vi "Functiongenerator_control.vi"(2 "error in (no error)":errorcluster, 3 "Data in":string="0 0.5 1000 0 0 2 0 0 0") -> (0 "error out (no error)":errorcluster, 1 "Data Out":string)   [LabVIEW 2011]
doc: "Function Generator VI\nControls a function generator."
uses:
  Server_Globals.vi
panel:
  in  "Duty Cycle High":dbl
  out "User waveform data":dbl[](array[numeric]) format="%.2f"
  in  "Burst count":i32=15
  in  "trigger source":T1(ring)=enum."External" caption="Trigger Source"
  in  "trigger mode":T2(ring)=enum."Stepped" caption="Trigger Mode"
  in  "Waveform":T3(ring)=enum."Square"
  out "Graph":dbl[](graph) caption="User waveform Graph"
  in  "Channel name":string="0"
  in  "Start phase":dbl format="%.2f"
  in  "DC Offset":dbl format="%.2f"
  in  "Amplitude":dbl=0.5 format="%.2f"
  in  "Frequency":dbl=10000.0 format="%.2f"
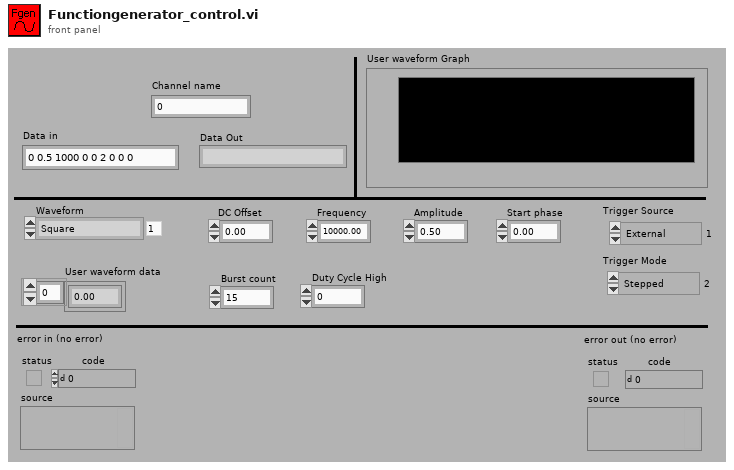
[diagram p1: front panel]
types:
  T1 = enum16{"Immediate", "External", "Software Trigger VI", "GPIB Get", "TTL0", "TTL1", "TTL2", "TTL3", "TTL4", "TTL5", "TTL6", "TTL7", "ECL0", "ECL1", "PXI Star", "RTSI 0", "RTSI 1", "RTSI 2", "RTSI 3", "RTSI 4", "RTSI 5", "RTSI 6"}
  T2 = enum16{"Single", "Continuous", "Stepped", "Burst"}
  T3 = enum16{"Sine", "Square", "Triangle", "Ramp up", "Ramp down", "DC", "Noise", "User Defined"}
  T4 = cluster{"I/O Settings":u64[], "Instrument Handle":cluster{"5402":refnum<k15>, " 5112":refnum<k15>, "4072":refnum<k15>, "USB":refnum<visa-resource-name>, "4110":refnum<k15>}, "Logfile":refnum<file>, "Log Level":i8, "Clear":i32[], "OS Set":cluster{"instrument handle out":refnum<k15>, "remaining string":string, "Settings":cluster{"Horizontal Conf.":cluster{"Min. Sample rate":dbl, "Reference position":dbl, "Record Length":i16}, "Channel A":cluster{"Enable":bool, "Vertical coupling":dbl, "Vertical range":dbl, "Vertical offset":dbl, "Probe attenuation":dbl}, "Channel B":cluster{"Enable":bool, "Vertical coupling":dbl, "Vertical range":dbl, "Vertical offset":dbl, "Probe attenuation":dbl}, "Trigger":cluster{"Source":enum8{"channel 1", "channel 2", "Imediate", "External trigger"}, "Slope":enum8{"Positive", "Negative"}, "Coupling":enum8{"AC", "DC"}, "Level":dbl, "Holdoff":dbl, "Delay":dbl, " Timeout":dbl, " Mode":enum8{"Normal", "Auto", "Auto Level"}}, "Measurements":cluster{"Measurement 1, Channel":enum8{"Channel 1", "Channel 2", "Channel 3", "Channel 4"}, "Measurement 1, Selection":u16, "Measurement 2, Channel":enum8{"Channel 1", "Channel 2", "Channel 3", "Channel 4"}, "Measurement 2,  Selection":u16, "Measurement 3, Channel":enum8{"Channel 1", "Channel 2", "Channel 3", "Channel 4"}, "Measurement 3, Selection 3":u16}}}, "DC Power Supply":cluster{"0":refnum<k15>, "1":refnum<k15>, "2":refnum<k15>, "3":refnum<k15>, "4":refnum<k15>}, "USB Interface":cluster{"0":refnum<visa-resource-name>, "1":refnum<visa-resource-name>, "2":refnum<visa-resource-name>, "3":refnum<visa-resource-name>, "4":refnum<visa-resource-name>}, "Function Generator":cluster{"0":refnum<k15>, "1":refnum<k15>, "2":refnum<k15>, "3":refnum<k15>, "4":refnum<k15>}, "Digital Multimeter":cluster{"0":refnum<k15>, "1":refnum<k15>, "2":refnum<k15>, "3":refnum<k15>, "4":refnum<k15>}, "Digital Osciliscope":cluster{"0":refnum<k15>, "1":refnum<k15>, "2":refnum<k15>, "3":refnum<k15>, "4":refnum<k15>}, "To M Server":string, "Adres":string[][], "Matrix version":string, "MD5":string, "Digital Multimeter Card 2":cluster{"0":string, "1":string, "2":string, "3":string, "4":string}}
  T5 = cluster{"0":refnum<k15>, "1":refnum<k15>, "2":refnum<k15>, "3":refnum<k15>, "4":refnum<k15>}
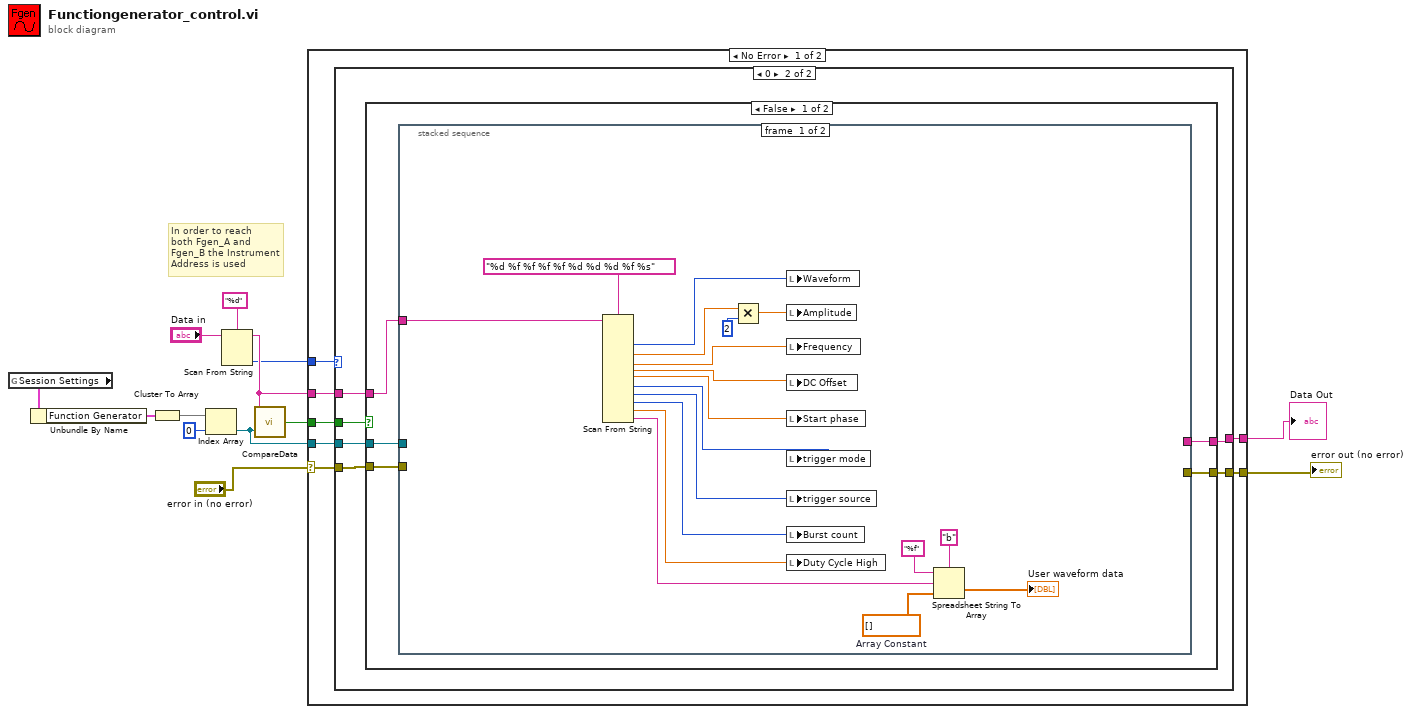
[diagram p0: block diagram]
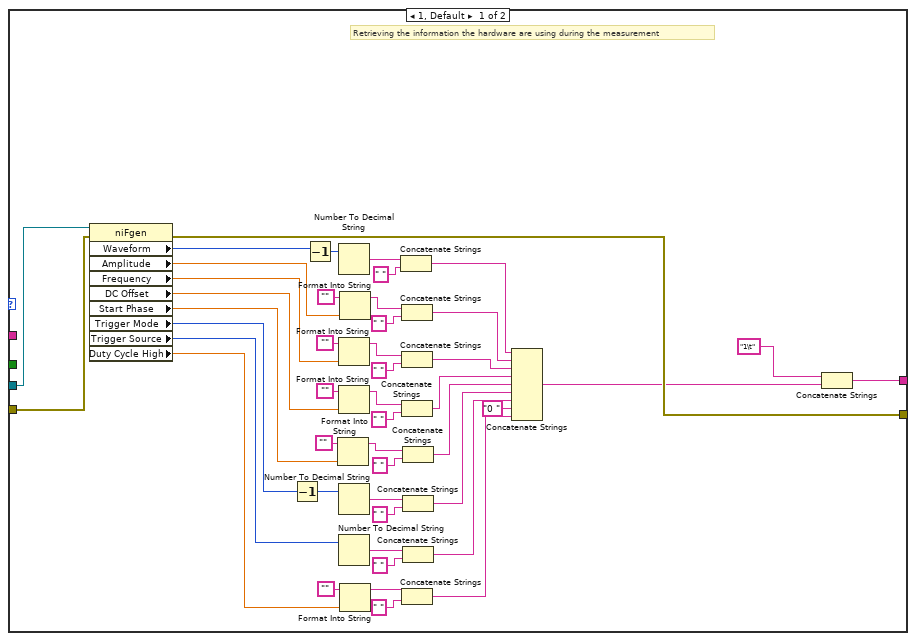
[diagram p2: hidden frame]
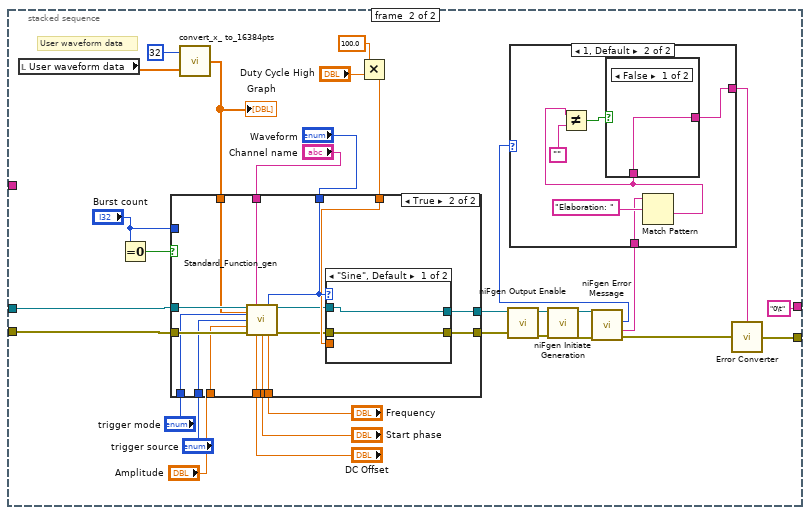
[diagram p3: hidden frame]
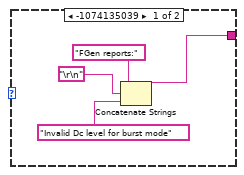
[diagram p4: hidden frame]
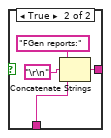
[diagram p5: hidden frame]
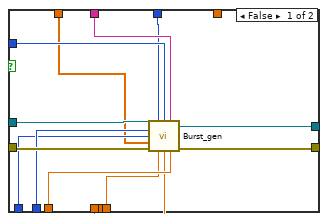
[diagram p6: hidden frame]
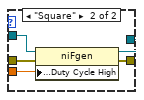
[diagram p7: hidden frame]
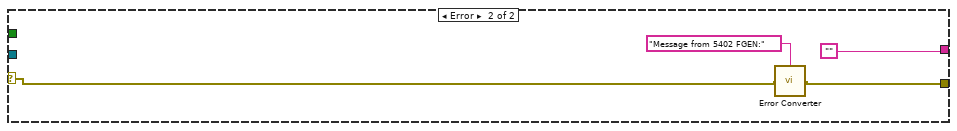
[diagram p9: hidden frame]
diagram:
  # "In order to reach \nboth Fgen_A and \nFgen_B the Instrument\nAddress is used"
  n1 = global read "Server_Globals.vi" "Session Settings"() -> (w5:T4)
  n2 = Unbundle By Name(w5) -> ("Function Generator"=w4:T5)
  n3 = Cluster To Array(cluster=w4) -> (array=w3:refnum<k15>[])
  n4 = Index Array(array=w3, index=0) -> (element=w1:refnum<k15>)
  n5 = Scan From String(format string="%d", input string="Data in") -> (remaining string=w10:string, output 1=w9:i32)  [unwired: 3 in, 2 out]
  n6 = call "CompareData.vi"("Que Name"=w1, "Data input"=w10) -> ("Same as before"=w13:bool)
  n7 = case shown="No Error" "error in (no error)" {
    selector: "error in (no error)" -> [w15 w181]
    tunnel: w13 -> [w20 _]
    tunnel: w1 -> [w19 _]
    tunnel: w10 -> [w18 _]
    tunnel: w9 -> [w17 _]
    tunnel: [w16 w180] -> w8
    tunnel: [w14 ""] -> w6
    frame No Error {
      n8 = case shown="0" w17 {
        tunnel: w20 -> [_ w72]
        tunnel: w18 -> [_ w71]
        tunnel: w19 -> [w29 w70]
        tunnel: w15 -> [w27 w69]
        tunnel: [w26 w68] -> w16
        tunnel: [w23 w67] -> w14
        frame 1, Default {
          # "Retrieving the information the hardware are using during the measurement"
          n9 = property class="niFgen"(reference=w29, error in=w27) -> (error out=w26:errorcluster, "Waveform"=w63:i32, "Amplitude"=w44:dbl, "Frequency"=w39:dbl, "DC Offset"=w36:dbl, "Start Phase"=w34:dbl, "Trigger Mode"=w24:i32, "Trigger Source"=w53:i32, "Duty Cycle High"=w30:dbl)  [unwired: 1 out]
          n10 = Decrement(x=w24) -> (x-1=w25:i32)
          n11 = Decrement(x=w63) -> (x-1=w66:i32)
          n12 = Format Into String(initial string="", w34) -> (resulting string=w33:string)  [unwired: 2 in, 1 out]
          n13 = Number To Decimal String(number=w66) -> (decimal integer string=w65:string)  [unwired: 1 in]
          n14 = Format Into String(initial string="", w39) -> (resulting string=w40:string)  [unwired: 2 in, 1 out]
          n15 = Format Into String(initial string="", w36) -> (resulting string=w37:string)  [unwired: 2 in, 1 out]
          n16 = Number To Decimal String(number=w25) -> (decimal integer string=w57:string)  [unwired: 1 in]
          n17 = Number To Decimal String(number=w53) -> (decimal integer string=w55:string)  [unwired: 1 in]
          n18 = Format Into String(initial string="", w44) -> (resulting string=w42:string)  [unwired: 2 in, 1 out]
          n19 = Format Into String(initial string="", w30) -> (resulting string=w31:string)  [unwired: 2 in, 1 out]
          n20 = Concatenate Strings(w65, " ") -> (w52:string)
          n21 = Concatenate Strings(w42, " ") -> (w51:string)
          n22 = Concatenate Strings(w40, " ") -> (w50:string)
          n23 = Concatenate Strings(w37, " ") -> (w49:string)
          n24 = Concatenate Strings(w31, " ") -> (w45:string)
          n25 = Concatenate Strings(w33, " ") -> (w48:string)
          n26 = Concatenate Strings(w57, " ") -> (w47:string)
          n27 = Concatenate Strings(w55, " ") -> (w46:string)
          n28 = Concatenate Strings(w52, w51, w50, w49, w48, w47, w46, "0 ", w45) -> (w22:string)
          n29 = Concatenate Strings("1\t", w22) -> (w23:string)
        }
        frame 0 {
          n30 = case shown="False" w72 {
            tunnel: w71 -> [w77 _]
            tunnel: w70 -> [w76 _]
            tunnel: w69 -> [w75 w178]
            tunnel: [w74 w178] -> w68
            tunnel: [w73 "0\t"] -> w67
            frame False {
              n31 = stacked-sequence {
                tunnel: w77 -> [w81 _]
                tunnel: w76 -> [_ w125]
                tunnel: w75 -> [_ w124]
                tunnel: [_ w123] -> w74
                tunnel: [_ "0\t"] -> w73
                frame #0 {
                  w94 = dbl[] []  # Array Constant
                  n32 = Scan From String(format string="%d %f %f %f %f %d %d %d %f %s" ("Format String"), input string=w81) -> (output 1=w90:i32, output 2=w83:dbl, output 3=w89:dbl, output 4=w88:dbl, output 5=w87:dbl, output 6=w86:i32, output 7=w85:i32, output 8=w80:i32, output 9=w78:dbl, output 10=w79:string)  [unwired: 12 in, 3 out]
                  n33 = Multiply(x=w83, y=2) -> (x*y=w84:dbl)
                  n34 = local write "Waveform"(w90) -> ()
                  n35 = local write "Amplitude"(w84) -> ()
                  n36 = local write "Frequency"(w89) -> ()
                  n37 = local write "DC Offset"(w88) -> ()
                  n38 = local write "Start phase"(w87) -> ()
                  n39 = local write "trigger mode"(w86) -> ()
                  n40 = local write "trigger source"(w85) -> ()
                  n41 = local write "Burst count"(w80) -> ()
                  n42 = local write "Duty Cycle High"(w78) -> ()
                  n43 = Spreadsheet String To Array(delimiter (Tab)="b", format string="%f", spreadsheet string=w79, array type (2D Dbl)=w94) -> (array=→"User waveform data":dbl[])
                }
                frame #1 {
                  # "User waveform data"
                  n44 = local read "User waveform data"() -> (w106:dbl[])
                  n45 = Equal To 0?(x="Burst count") -> (x = 0?=w108:bool)
                  n46 = call "convert_x_ to_16384pts.vi"("User waveform data"=w106, "Convert_Factor"=32) -> ("Waveform out"=w96:dbl[])
                  "Graph" <- w96
                  n47 = Multiply(x=100.0, y="Duty Cycle High") -> (x*y=w100:dbl)
                  n48 = case shown="True" w108 {
                    tunnel: w125 -> [w153 w169]
                    tunnel: w124 -> [w152 w168]
                    tunnel: [w151 w156] -> w118
                    tunnel: [w150 w157] -> w117
                    tunnel: "Channel name" -> [w149 w167]
                    tunnel: "trigger mode" -> [w147 w166]
                    tunnel: "trigger source" -> [w148 w165]
                    tunnel: "Amplitude" -> [w146 w164]
                    tunnel: "Start phase" -> [_ w160]
                    tunnel: "DC Offset" -> [w145 w162]
                    tunnel: "Frequency" -> [w144 w161]
                    tunnel: "Waveform" -> [w142 w159]
                    tunnel: w96 -> [w141 w163]
                    tunnel: "Burst count" -> [w143 _]
                    tunnel: w100 -> [_ w158]
                    frame False {
                      n49 = call "Burst_gen.vi"("Instrument handle"=w153, "Waveform in"=w142, "Burst count"=w143, "Channel name"=w149, "Trigger source"=w148, "Trigger mode"=w147, "User defined waveform"=w141, "error in (no error)"=w152, "Frequency"=w144, "DC Offset"=w145, "Amplitude"=w146) -> ("Instrument handle out"=w150:refnum<k15>, "error out"=w151:errorcluster)  [unwired: 3 in]
                    }
                    frame True {
                      n50 = call "Standard_Function_gen.vi"("Instrument handle in"=w169, "Channel name"=w167, "User defined waveform"=w163, "Waveform"=w159, "Trigger mode"=w166, "Trigger source"=w165, "Amplitude"=w164, "error in (no error)"=w168, "DC Offset"=w162, "Start phase"=w160, "Frequency"=w161) -> ("Instrument handle out"=w155:refnum<k15>, "error out"=w154:errorcluster)  [unwired: 3 in]
                      n51 = case shown="\"Sine\", Default" w159 {
                        tunnel: w158 -> [_ w176]
                        tunnel: [w171 w175] -> w157
                        tunnel: [w170 w174] -> w156
                        tunnel: w155 -> [w171 w173]
                        tunnel: w154 -> [w170 w172]
                        frame "Sine", Default {
                        }
                        frame "Square" {
                          n52 = property class="niFgen"(reference=w173, error in=w172, "Standard Function Output:Duty Cycle High"=w176) -> (reference out=w175:refnum<k15>, error out=w174:errorcluster)
                        }
                      }
                    }
                  }
                  n53 = call <instrlib>:"niFgen Output Enable.vi"("error in (no error)"=w118, "Instrument Handle"=w117) -> ("error out"=w121:errorcluster, "Instrument Handle Out"=w122:refnum<k15>)  [unwired: 8 in]
                  n54 = call <instrlib>:"niFgen Initiate Generation.vi"("error in (no error)"=w121, "Instrument Handle"=w122) -> ("error out"=w119:errorcluster, "Instrument Handle Out"=w120:refnum<k15>)  [unwired: 8 in]
                  n55 = call <instrlib>:"niFgen Error Message.vi"("error in (no error)"=w119, "Instrument Handle"=w120) -> ("error out"=w98:errorcluster, "Error Message"=w107:string, "Error Code"=w104:i32)  [unwired: 6 in, 1 out]
                  n56 = case shown="1, Default" w104 {
                    tunnel: w107 -> [_ w134]
                    tunnel: [w126 w132] -> w103
                    frame -1074135039 {
                      n57 = Concatenate Strings("FGen reports:", "\r\n", "Invalid Dc level for burst mode") -> (w126:string)
                    }
                    frame 1, Default {
                      n58 = Match Pattern(string=w134, regular expression="Elaboration: ") -> (after substring=w130:string)  [unwired: 1 in, 3 out]
                      n59 = Not Equal?(x=w130, y="") -> (x != y?=w131:bool)
                      n60 = case shown="False" w131 {
                        tunnel: [w136 w138] -> w132
                        tunnel: w130 -> [w136 w137]
                        frame False {
                        }
                        frame True {
                          n61 = Concatenate Strings("FGen reports:", "\r\n", w137) -> (w138:string)
                        }
                      }
                    }
                  }
                  n62 = call "Error Converter.vi"("error in (no error)"=w98, "String to add to error message"=w103) -> ("error out (no error)"=w123:errorcluster)
                }
              }
            }
            frame True {
            }
          }
        }
      }
    }
    frame Error {
      n63 = call "Error Converter.vi"("error in (no error)"=w181, "String to add to error message"="Message from 5402 FGEN:" ("String to add message")) -> ("error out (no error)"=w180:errorcluster)
    }
  }
  "error out (no error)" <- w8
  "Data Out" <- w6
